vi "Read CCDF (Probability and Power Level).vi"(8 "error in (no error)":errorcluster, 9 "Power Level (0)":dbl, 10 "Probability (0)":dbl, 11 "VISA resource name":refnum<visa-resource-name>) -> (0 "error out":errorcluster, 1 "Probability at Specified Power Level":dbl, 2 "Power Level at Specified Probability":dbl, 3 "VISA resource name out":refnum<visa-resource-name>, 4 "Probability Values Array":dbl[](array[numeric]))   [LabVIEW 2014, in "Agilent U2000 Series.lvlib"]
doc: "Returns probability values and power levels.\n\nNote:\nThis VI is only applicable when the NORMal or DOUBle measurement speed\nsetting is chosen.\n\nThis VI is not applicable for U2040 X-Series."
uses:
  Agilent U2000 Series.lvlib
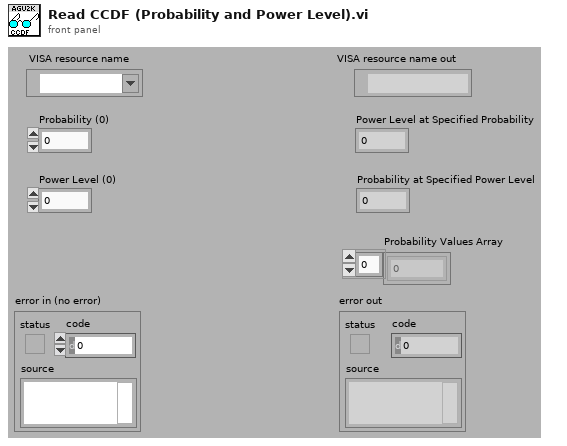
[diagram p1: front panel]
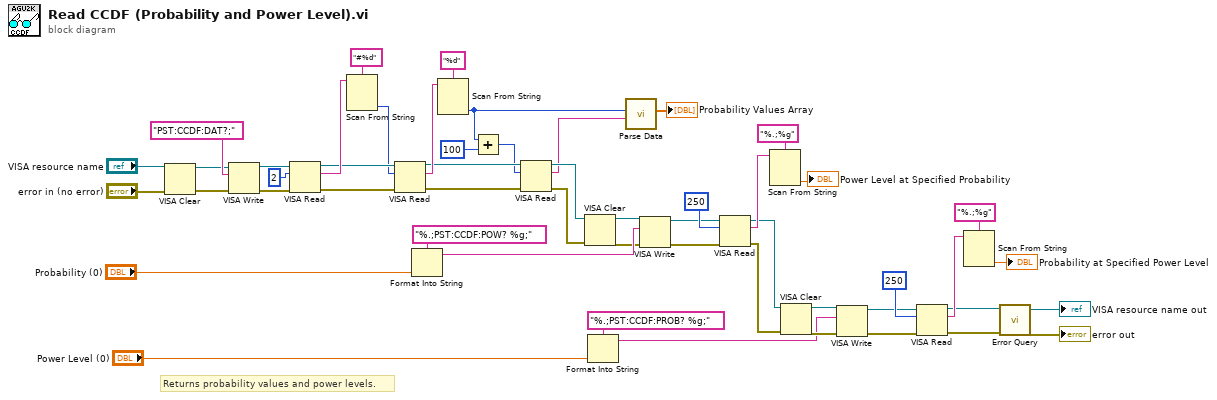
[diagram p0: block diagram]
diagram:
  # "Returns probability values and power levels."
  n1 = VISA Clear(VISA resource name="VISA resource name", error in (no error)="error in (no error)") -> (VISA resource name out=w49:refnum<visa-resource-name>, error out=w48:errorcluster)
  n2 = VISA Write(VISA resource name=w49, write buffer="PST:CCDF:DAT?;", error in (no error)=w48) -> (VISA resource name out=w13:refnum<visa-resource-name>, error out=w12:errorcluster)  [unwired: 1 out]
  n3 = VISA Read(VISA resource name=w13, byte count=u32 2, error in (no error)=w12) -> (VISA resource name out=w22:refnum<visa-resource-name>, read buffer=w24:string, error out=w21:errorcluster)  [unwired: 1 out]
  n4 = Scan From String(format string="#%d", input string=w24) -> (output 1=w20:i32)  [unwired: 2 in, 4 out]
  n5 = VISA Read(VISA resource name=w22, byte count=w20, error in (no error)=w21) -> (VISA resource name out=w17:refnum<visa-resource-name>, read buffer=w18:string, error out=w16:errorcluster)  [unwired: 1 out]
  n6 = Format Into String(format string="%.;PST:CCDF:POW? %g;", "Probability (0)") -> (resulting string=w45:string)  [unwired: 2 in, 1 out]
  n7 = Scan From String(format string="%d", input string=w18) -> (output 1=w2:i32)  [unwired: 2 in, 4 out]
  n8 = Add(x=w2, y=100) -> (x+y=w14:i32)
  n9 = VISA Read(VISA resource name=w17, byte count=w14, error in (no error)=w16) -> (VISA resource name out=w10:refnum<visa-resource-name>, read buffer=w3:string, error out=w11:errorcluster)  [unwired: 1 out]
  n10 = VISA Clear(VISA resource name=w10, error in (no error)=w11) -> (VISA resource name out=w43:refnum<visa-resource-name>, error out=w44:errorcluster)
  n11 = Format Into String(format string="%.;PST:CCDF:PROB? %g;", "Power Level (0)") -> (resulting string=w28:string)  [unwired: 2 in, 1 out]
  n12 = call "Parse Data.vi"("Read Buffer"=w3, "Data Length"=w2) -> ("Output Data Array"=→"Probability Values Array":dbl[])  [unwired: 9 out]
  n13 = VISA Write(VISA resource name=w43, write buffer=w45, error in (no error)=w44) -> (VISA resource name out=w41:refnum<visa-resource-name>, error out=w40:errorcluster)  [unwired: 1 out]
  n14 = VISA Read(VISA resource name=w41, byte count=u32 250, error in (no error)=w40) -> (VISA resource name out=w29:refnum<visa-resource-name>, read buffer=w38:string, error out=w30:errorcluster)  [unwired: 1 out]
  n15 = Scan From String(format string="%.;%g", input string=w38) -> (output 1=→"Power Level at Specified Probability":dbl)  [unwired: 2 in, 4 out]
  n16 = VISA Clear(VISA resource name=w29, error in (no error)=w30) -> (VISA resource name out=w35:refnum<visa-resource-name>, error out=w36:errorcluster)
  n17 = VISA Write(VISA resource name=w35, write buffer=w28, error in (no error)=w36) -> (VISA resource name out=w33:refnum<visa-resource-name>, error out=w32:errorcluster)  [unwired: 1 out]
  n18 = VISA Read(VISA resource name=w33, byte count=u32 250, error in (no error)=w32) -> (VISA resource name out=w6:refnum<visa-resource-name>, read buffer=w31:string, error out=w4:errorcluster)  [unwired: 1 out]
  n19 = Scan From String(format string="%.;%g", input string=w31) -> (output 1=→"Probability at Specified Power Level":dbl)  [unwired: 2 in, 4 out]
  n20 = call "Error Query.vi"("error in (no error)"=w4, "VISA resource name"=w6) -> ("error out"=→"error out":errorcluster, "VISA resource name out"=→"VISA resource name out":refnum<visa-resource-name>)  [unwired: 8 out]
